vi "Bool Set Reset.vi"(9 "clear":bool, 10 "set":bool) -> (2 "out":bool)   [LabVIEW 2013, in "Engine Simulation Toolkit.lvlib"]
uses:
  Engine Simulation Toolkit.lvlib
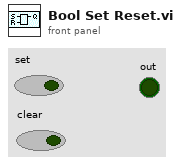
[diagram p1: front panel]
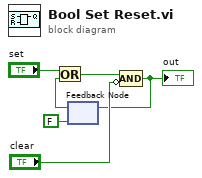
[diagram p0: block diagram]
diagram:
  n1 = feedback #1(FALSE) -> (w1:bool)
  n2 = Or(x="set", y=w1) -> (x .or. y?=w4:bool)
  n3 = Compound Arithmetic op=AND(w4, invert "clear") -> (w3:bool)
  "out" <- w3
  n4 = feedback-in #1(w3) -> ()
